vi "FTW-JSON-Object-GetElement-DBL.vi"(0 "JSON Object":refnum<data-value>, 5 "Key":string, 7 "Default Value":dbl=nan, 9 "Remove Value":bool, 11 "error in":errorcluster) -> (4 "JSON Object out":refnum<data-value>, 6 "JSON Element Type":T1, 8 "Value":dbl, 15 "error out":errorcluster)   [LabVIEW 2015]
uses:
  core/FTW-JSON-Core-Structure.ctl
  FTW-JSON-Type.ctl
  core/FTW-JSON-Core-Type.ctl
panel:
  # "Inputs"
  # "Outputs"
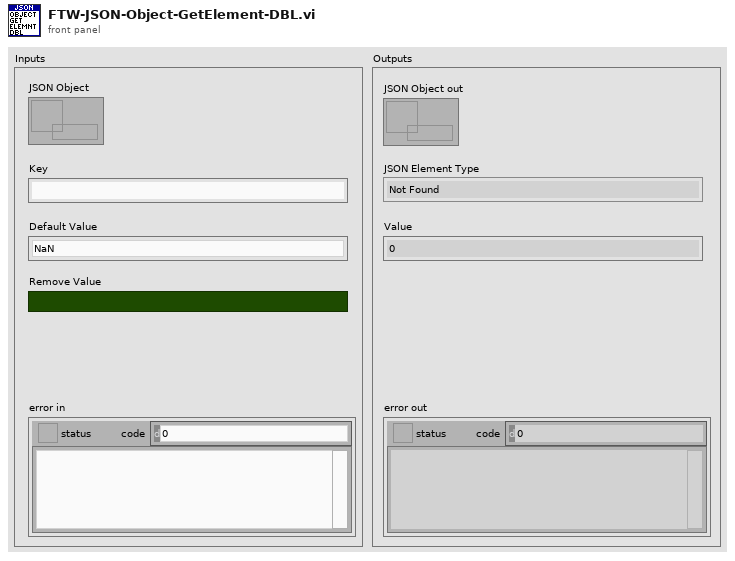
[diagram p1: front panel]
types:
  T1 = typedef "FTW-JSON-Type.ctl" = enum8{"Not Found", "Object", "Array", "String", "Number", "Boolean", "null"}
  T2 = typedef "FTW-JSON-Core-Type.ctl" = enum8{"Object", "Array", "String", "Integer", "Floating Point", "true", "false", "null", "undefined"}
  T3 = typedef "FTW-JSON-Core-Structure.ctl" = cluster{"JSON Object":i64, "Encoding Flags":i64, "Decoding Flags":i64}
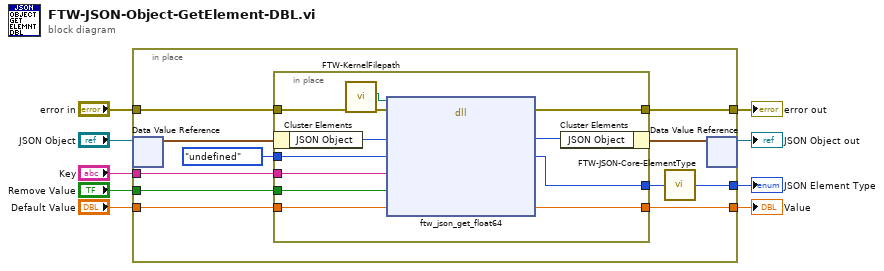
[diagram p0: block diagram]
diagram:
  n1 = in-place {
    in-place-border: "error in" -> [w20]
    in-place-border: "Key" -> [w19]
    in-place-border: [w11] -> w2
    in-place-border: [w17] -> w4
    in-place-border: "Default Value" -> [w18]
    in-place-border: "Remove Value" -> [w13]
    in-place-border: [w10] -> w1
    n2 = in-place-dvr #1("JSON Object") -> (w16:T3)  [unwired: 1 out]
    n3 = in-place {
      in-place-border: w20 -> [w23]
      in-place-border: w19 -> [w32]
      in-place-border: w18 -> [w31]
      in-place-border: [w30] -> w17
      in-place-border: [w29] -> w11
      in-place-border: [w28] -> w12
      in-place-border: FTW-JSON-Core-Type."undefined" ("JSON Type") -> [w27]
      in-place-border: w13 -> [w24]
      n4 = in-place-cluster #2(w16) -> ("JSON Object"=w26:i64)
      n5 = call "FTW-KernelFilepath.vi"("error in"=w23) -> ("error out"=w22:errorcluster, "Library Filepath"=w21:path)  [unwired: 8 in, 1 out]
      n6 = dll-call lib="?" fn="ftw_json_get_float64"(path in=w21, error in=w22, "JSON Object"=w26, "Type"=w27, "Element Key"=w32, "Remove?"=w24, "Value"=w31) -> (error out=w29:errorcluster, "JSON Object"=w25:i64, "Type"=w28:T2, "Value"=w30:dbl)  [unwired: 4 in, 1 out]
      n7 = in-place-cluster #2("JSON Object"=w25) -> (w15:T3)
    }
    n8 = call "FTW-JSON-Core-ElementType.vi"("Core Type"=w12) -> ("JSON Element Type"=w10:T1)
    n9 = in-place-dvr #1(w15) -> (→"JSON Object out":refnum<data-value>)  [unwired: 1 out]
  }
  "error out" <- w2
  "Value" <- w4
  "JSON Element Type" <- w1
